vi "ReadAlarmsConfiguration.vi"(8 "Error In":errorcluster, 11 "ABLE Config File Ref In":T2) -> (0 "Error Out":errorcluster, 2 "Alarms Configuration":T1, 3 "ABLE Config File Ref Out":T2)   [LabVIEW 2012]
uses:
  <vilib>/Utility/config.llb/Config Data RefNum.ctl
  AlarmsConfiguration.ctl
  <vilib>/Utility/config.llb/Read Key (Path).vi
  <vilib>/Utility/config.llb/Read Key (Double).vi
  <vilib>/Utility/config.llb/NI_LVConfig.lvlib
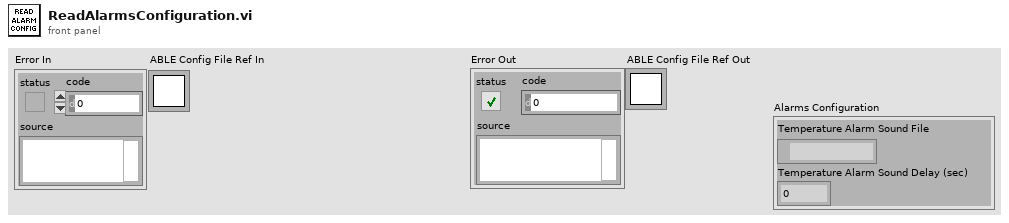
[diagram p1: front panel]
types:
  T1 = typedef "AlarmsConfiguration.ctl" = cluster{"Temperature Alarm Sound File":path, "Temperature Alarm Sound Delay (sec)":dbl}
  T2 = typedef "NI_LVConfig.lvlib/Config Data RefNum.ctl" = refnum<k1>
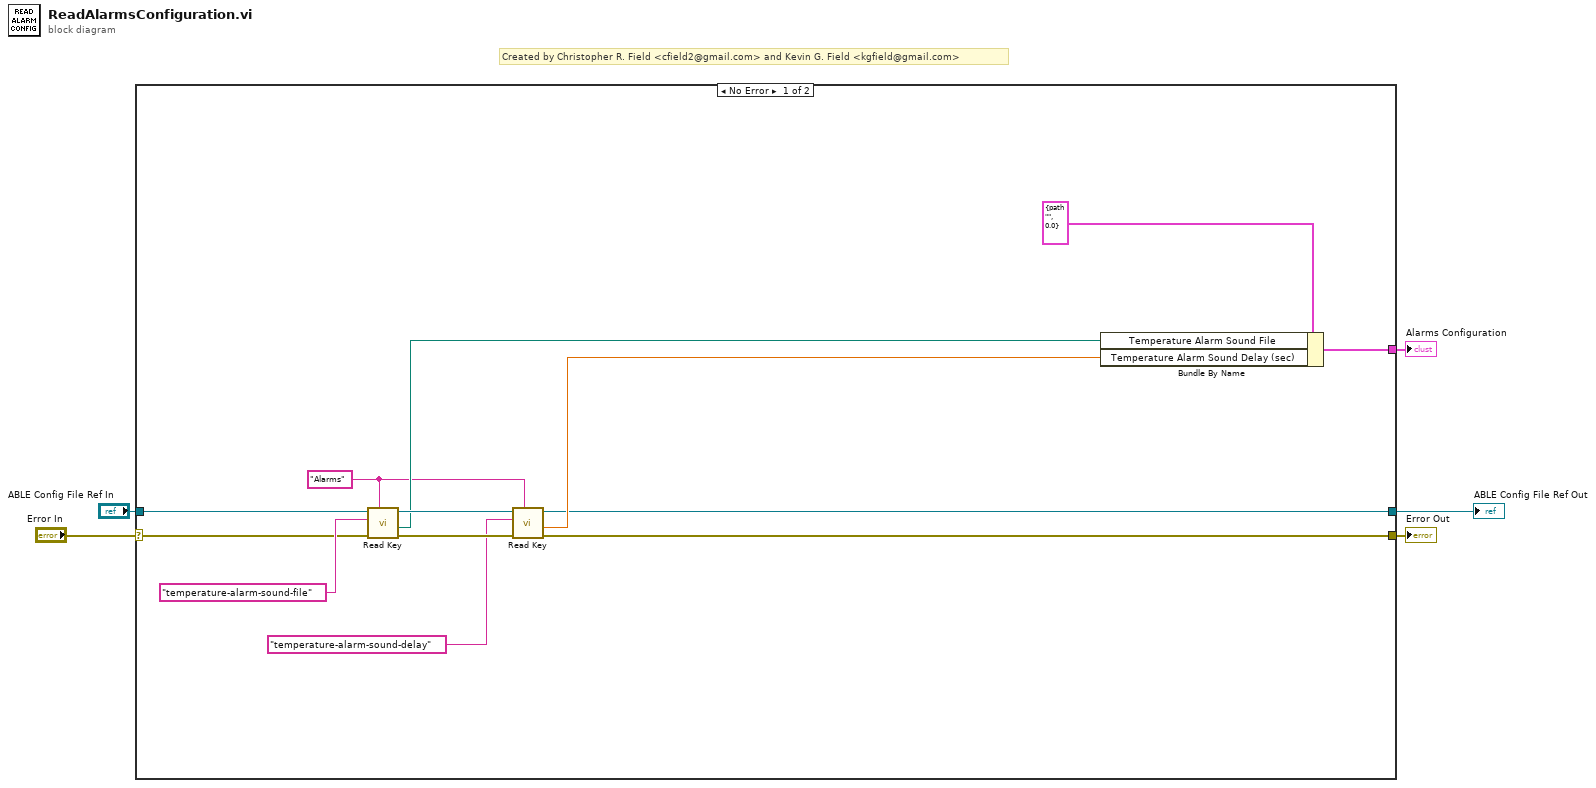
[diagram p0: block diagram]
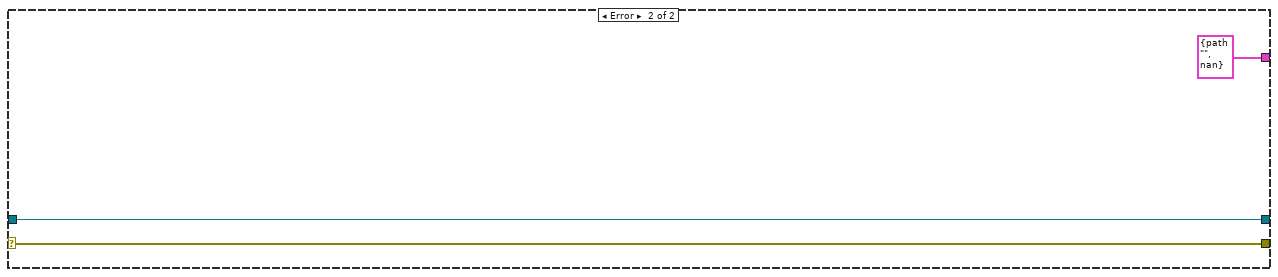
[diagram p2: hidden frame]
diagram:
  # "Created by Christopher R. Field <cfield2@gmail.com> and Kevin G. Field <kgfield@gmail.com>"
  n1 = case shown="No Error" "Error In" {
    selector: "Error In" -> [w14 w20]
    tunnel: [w6 w20] -> w4
    tunnel: [w7 w21] -> w3
    tunnel: "ABLE Config File Ref In" -> [w13 w21]
    tunnel: [w10 T1 {"Temperature Alarm Sound File"=path "", "Temperature Alarm Sound Delay (sec)"=nan} ("Alarms Configuration")] -> w1
    frame No Error {
      w8 = "Alarms" ("section")
      n2 = call-poly <vilib>:"Read Key.vi"("section"=w8, "error in (no error)"=w14, "key"="temperature-alarm-sound-file", "refnum"=w13) -> ("error out"=w16:errorcluster, "value"=w12:path, "refnum out"=w17:T2)  [unwired: 4 in, 1 out]
      n3 = call-poly <vilib>:"Read Key.vi"("section"=w8, "error in (no error)"=w16, "key"="temperature-alarm-sound-delay", "refnum"=w17) -> ("error out"=w6:errorcluster, "value"=w9:dbl, "refnum out"=w7:T2)  [unwired: 4 in, 1 out]
      n4 = Bundle By Name(cluster=T1 {"Temperature Alarm Sound File"=path "", "Temperature Alarm Sound Delay (sec)"=0.0} ("Alarms Configuration"), "Temperature Alarm Sound File"=w12, "Temperature Alarm Sound Delay (sec)"=w9) -> (w10:T1)
    }
    frame Error {
    }
  }
  "Error Out" <- w4
  "ABLE Config File Ref Out" <- w3
  "Alarms Configuration" <- w1
